vi "ViHandler.RegisterVi.vi"(8 "error in (no error)":errorcluster, 10 "ViInfo":T1, 11 "ViHandler in":refnum<class "ViHandler.lvclass">) -> (0 "error out":errorcluster, 3 "ViHandler out":refnum<class "ViHandler.lvclass">)   [LabVIEW 2016, in "ViHandler.lvclass"]
uses:
  ViHandler.lvclass
  ViHandler.ViInfo.ctl
  ViHandler.lvclass/ViHandler.ctl
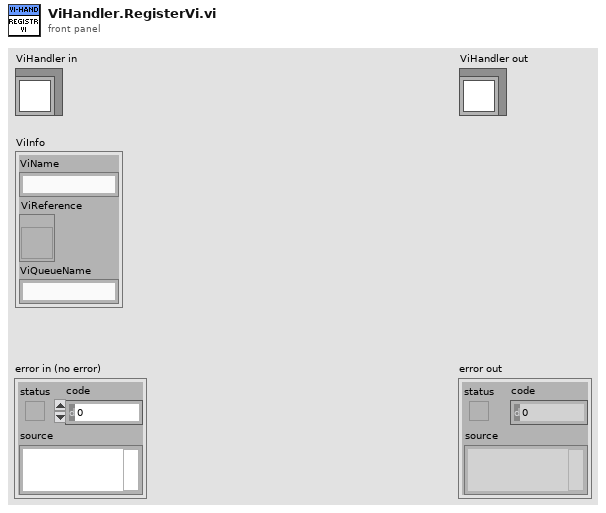
[diagram p1: front panel]
types:
  T1 = typedef "ViHandler.lvclass/ViHandler.ViInfo.ctl" = cluster{"ViName":string, "ViReference":refnum<vi>, "ViQueueName":string}
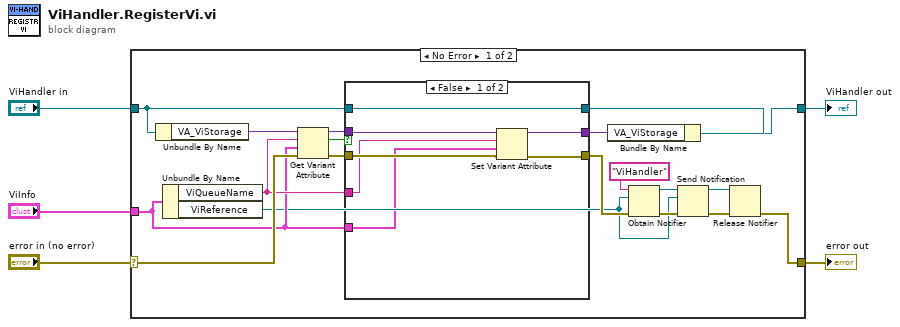
[diagram p0: block diagram]
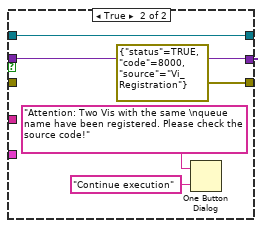
[diagram p2: hidden frame]
diagram:
  n1 = case shown="No Error" "error in (no error)" {
    selector: "error in (no error)" -> [w23 w38]
    tunnel: [w10 w38] -> w4
    tunnel: [w15 w37] -> w2
    tunnel: "ViHandler in" -> [w21 w37]
    tunnel: "ViInfo" -> [w16 _]
    frame No Error {
      n2 = Unbundle By Name(w21) -> ("VA_ViStorage"=w24:variant)
      n3 = Unbundle By Name(w16) -> ("ViQueueName"=w17:string, "ViReference"=w6:refnum<vi>)
      n4 = Get Variant Attribute(Variant=w24, name=w17, default value (empty Variant)=w16, error in=w23) -> (duplicate Variant=w19:variant, found=w22:bool, error out=w18:errorcluster)  [unwired: 1 out]
      n5 = case shown="False" w22 {
        tunnel: w21 -> [w31 w36]
        tunnel: [w31 w36] -> w20
        tunnel: w19 -> [w29 w32]
        tunnel: w18 -> [w30 _]
        tunnel: [w26 errorcluster {"status"=TRUE, "code"=8000, "source"="Vi_Registration"} ("error out")] -> w13
        tunnel: w17 -> [w28 _]
        tunnel: w16 -> [w27 _]
        tunnel: [w25 w32] -> w14
        frame False {
          n6 = Set Variant Attribute(Variant=w29, name=w28, value=w27, error in=w30) -> (Variant out=w25:variant, error out=w26:errorcluster)  [unwired: 1 out]
        }
        frame True {
          n7 = One Button Dialog(message="Attention: Two Vis with the same \nqueue name have been registered. Please check the source code!", button name ("OK")="Continue execution") -> ()  [unwired: 1 out]
        }
      }
      n8 = Bundle By Name(cluster=w20, "VA_ViStorage"=w14) -> (w15:refnum<class "ViHandler.lvclass">)
      n9 = Obtain Notifier(name (unnamed)="ViHandler", notification data type=w6, error in (no error)=w13) -> (notifier out=w8:refnum<notifier>, error out=w11:errorcluster)  [unwired: 1 in, 1 out]
      n10 = Send Notification(notification=w6, notifier=w8, error in (no error)=w11) -> (notifier out=w9:refnum<notifier>, error out=w12:errorcluster)
      n11 = Release Notifier(notifier=w9, error in (no error)=w12) -> (error out=w10:errorcluster)  [unwired: 1 in, 2 out]
    }
    frame Error {
    }
  }
  "error out" <- w4
  "ViHandler out" <- w2
